vi "Get All Library VI Data.vi"(8 "error in":errorcluster, 11 "Lvlib Path":path) -> (0 "error out":errorcluster, 3 "Item Data":refnum<class "Item.lvclass">[](array[class]))   [LabVIEW 2020, in "VI Properties Editor.lvlib"]
doc: "Gets all VI data from a library located at <B>Path</B>."
uses:
  VI Properties Editor.lvlib
  Classes/Item/Item.lvclass
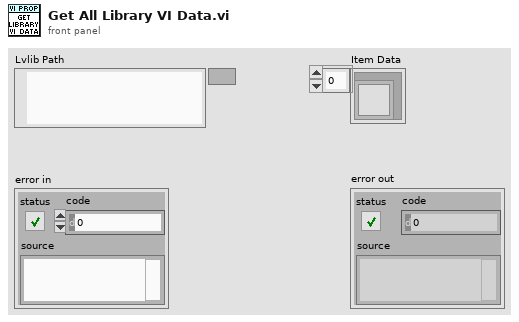
[diagram p1: front panel]
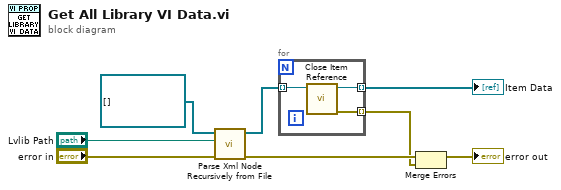
[diagram p0: block diagram]
diagram:
  n1 = call "Parse Xml Node Recursively from File.vi"("error in"="error in", "Path to XML document"="Lvlib Path", "Item Data"=refnum<class "Item.lvclass">[] []) -> ("error out"=w6:errorcluster, "Item Data out"=w2:refnum<class "Item.lvclass">[])  [unwired: 7 in]
  n2 = for {
    tunnel: [w11] -> w5 mode=indexing
    tunnel: w2 -> [w10] mode=indexing
    tunnel: [w9] -> w1 mode=indexing
    n3 = call-dynamic "Close Item Reference.vi"("Item in"=w10) -> ("error out"=w11:errorcluster, "Item out"=w9:refnum<class "Item.lvclass">)  [unwired: 9 in]
  }
  "Item Data" <- w1
  n4 = Merge Errors(w6, w5) -> (→"error out":errorcluster)
